vi "Operation UI.vi"(0 "Divide in":refnum<class "Divide.lvclass">, 5 "A":dbl, 7 "B":dbl, 9 "Calculate":bool, 11 "Error In":errorcluster, 12 "Stop":refnum<user-event>, 13 "Class Data":refnum<user-event>) -> (4 "Divide out":refnum<class "Divide.lvclass">, 6 "C":dbl, 15 "Error Out":errorcluster)   [LabVIEW 2023, in "Divide.lvclass"]
doc: "The VI contains the addition operation UI that accepts two input numbers and performs division operation and displays the output when user clicks calculate button"
uses:
  Divide.lvclass
  C:/Users/Ancy.Augustin/Downloads/LVOOPS DVR/LVOOPS DVR/Classes/Arithemtic Operation/Arithemetic Operation.lvclass
  Arithemtic Operation/Arithemetic Operation.lvclass
  Typedef/User Event Operations.ctl
panel:
  # "DIVISION"
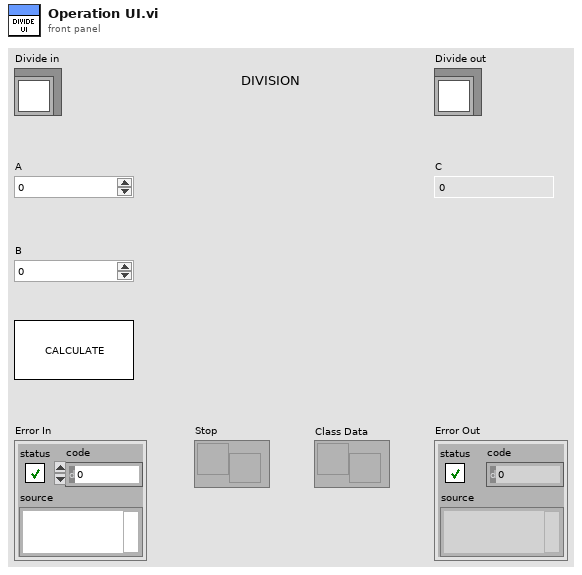
[diagram p1: front panel]
types:
  T1 = typedef "User Event Operations.ctl" = enum16{"Obtain", "Generate", "Release"}
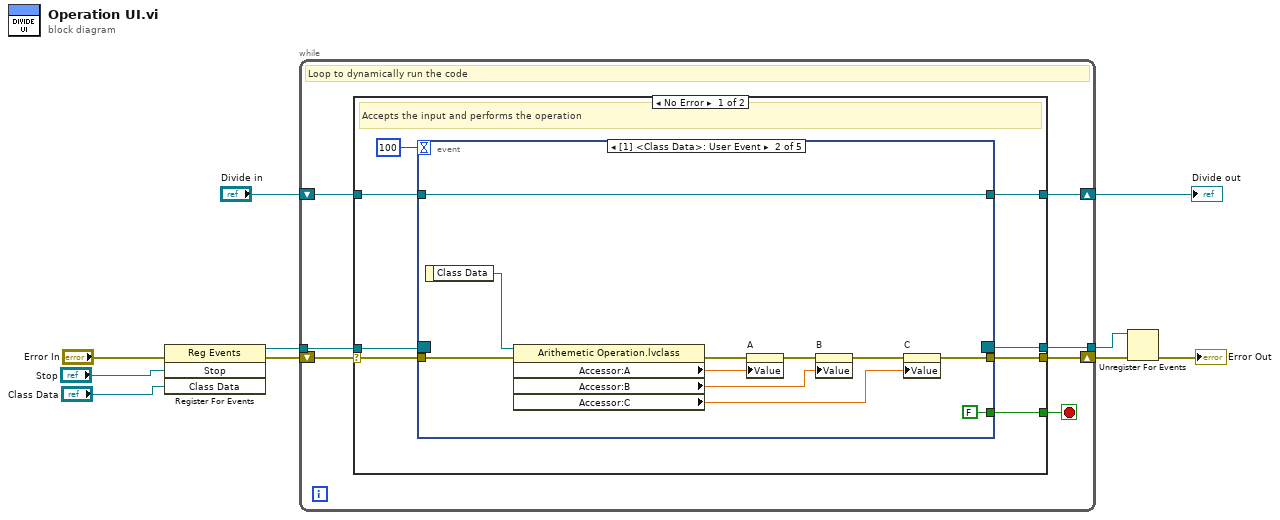
[diagram p0: block diagram]
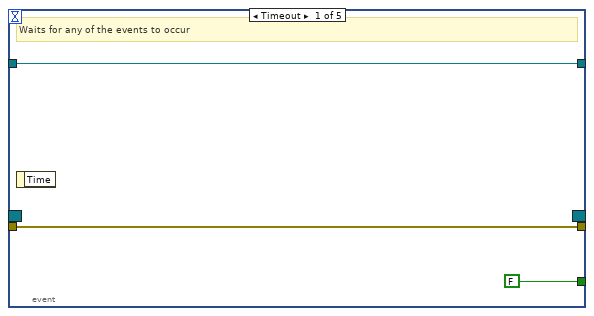
[diagram p2: hidden frame]
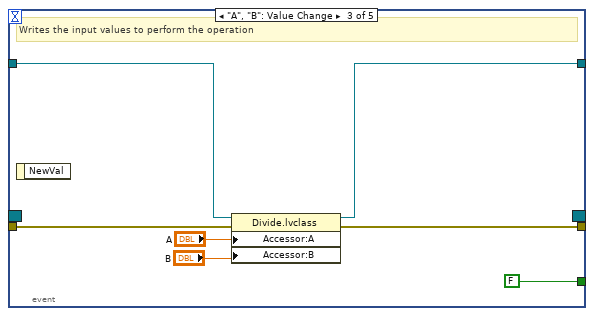
[diagram p3: hidden frame]
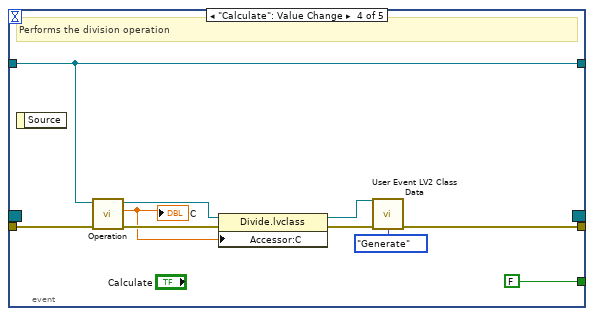
[diagram p4: hidden frame]
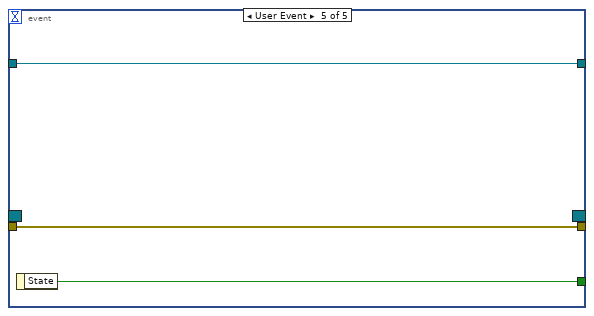
[diagram p5: hidden frame]
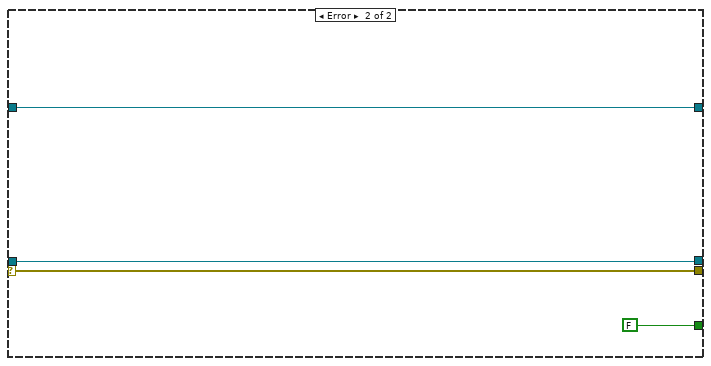
[diagram p6: hidden frame]
diagram:
  n1 = register-events(error in="Error In", "Stop", "Class Data") -> (reference out=w7:refnum<event-registration>, error out=w8:errorcluster)  [unwired: 1 in]
  n2 = while {
    shift-right: [w16] -> w10
    shift-left: w8 -> [w17]
    shift-right: [w14] -> w3
    shift-left: "Divide in" -> [w15]
    tunnel: w7 -> [w13]
    tunnel: [w12] -> w5
    stop <- w11 stop-if-true
    # "Loop to dynamically run the code"
    n3 = case shown="No Error" w17 {
      selector: w17 -> [w23 w63]
      tunnel: [w22 w63] -> w16
      tunnel: [w24 w62] -> w14
      tunnel: w15 -> [w25 w62]
      tunnel: w13 -> [w20 w61]
      tunnel: [w19 w61] -> w12
      tunnel: [w18 FALSE] -> w11
      frame No Error {
        # "Accepts the input and performs the operation"
        n4 = event shown="[1] <Class Data>: User Event" {
          selector: w20 -> [_ _ _ _ _]
          dyn-events: [_ _ _ _ _] -> w19
          timeout: 100 -> [_ _ _ _ _]
          tunnel: [w28 w39 w41 w52 w59] -> w24
          tunnel: w25 -> [w28 w39 w44 w52 w59]
          tunnel: w23 -> [w27 w38 w46 w56 w58]
          tunnel: [w27 w33 w45 w53 w58] -> w22
          tunnel: [FALSE FALSE FALSE FALSE w57] -> w18
          event Timeout {
            # "Waits for any of the events to occur"
            n5 = event-data() -> ()  [unwired: 1 in, 1 out]
          }
          event User Event {
            n6 = event-data() -> ("Class Data"=w36:refnum<class "Arithemetic Operation.lvclass">)  [unwired: 1 in]
            n7 = property class="Arithemetic Operation.lvclass"(reference=w36, error in=w38) -> (error out=w37:errorcluster, "Accessor:A"=w31:dbl, "Accessor:B"=w30:dbl, "Accessor:C"=w29:dbl)  [unwired: 1 out]
            n8 = property on="A" class="DigNum (strict)"(error in=w37, "Value"=w31) -> (error out=w35:errorcluster)  [unwired: 1 in, 1 out]
            n9 = property on="B" class="DigNum (strict)"(error in=w35, "Value"=w30) -> (error out=w34:errorcluster)  [unwired: 1 in, 1 out]
            n10 = property on="C" class="DigNum (strict)"(error in=w34, "Value"=w29) -> (error out=w33:errorcluster)  [unwired: 1 in, 1 out]
          }
          event "A", "B": Value Change {
            # "Writes the input values to perform the operation"
            n11 = event-data() -> ()  [unwired: 1 in, 1 out]
            n12 = property class="Divide.lvclass"(reference=w44, error in=w46, "Accessor:A"="A", "Accessor:B"="B") -> (reference out=w41:refnum<class "Divide.lvclass">, error out=w45:errorcluster)
          }
          event "Calculate": Value Change {
            # "Performs the division operation"
            n13 = event-data() -> ()  [unwired: 1 in, 1 out]
            n14 = call-dynamic "Operation.vi"("Error In"=w56, "Divide In"=w52) -> ("Error Out"=w55:errorcluster, "C"=w49:dbl, "Divide Out"=w50:refnum<class "Divide.lvclass">)  [unwired: 7 in]
            "C" <- w49
            n15 = property class="Divide.lvclass"(reference=w50, error in=w55, "Accessor:C"=w49) -> (reference out=w48:refnum<class "Divide.lvclass">, error out=w51:errorcluster)
            n16 = call "User Event LV2 Class Data.vi"("Class Data"=w48, "Error In"=w51, "Operation"=User_Event_Operations."Generate") -> ("Error Out"=w53:errorcluster)  [unwired: 11 in, 1 out]
          }
          event User Event {
            n17 = event-data() -> ("State"=w57:bool)  [unwired: 1 in]
          }
        }
      }
      frame Error {
      }
    }
  }
  "Divide out" <- w3
  n18 = Unregister For Events(event registration refnum=w5, error in=w10) -> (error out=→"Error Out":errorcluster)
